vi "Read Cooler Enqueuer.vi"(11 "Cooler Controller":refnum<class "Cooler Controller.lvclass">) -> (2 "Cooler Enqueuer":refnum<class "Message Enqueuer.lvclass">)   [LabVIEW 2018, in "Cooler Controller.lvlib" / "Cooler Controller.lvclass"]
doc: "This VI reads what cooler the controller is controlling. This VI may return a Not A Refnum enqueuer because there is no guarantee that the controller is in control of any cooler."
uses:
  Cooler Controller.lvclass
  <vilib>/ActorFramework/Message Enqueuer/Message Enqueuer.lvclass
  Cooler Controller.lvclass/Cooler Controller.ctl
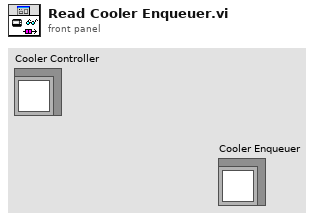
[diagram p1: front panel]
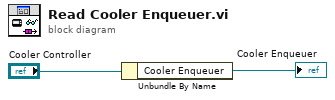
[diagram p0: block diagram]
diagram:
  n1 = Unbundle By Name("Cooler Controller") -> ("Cooler Enqueuer"=→"Cooler Enqueuer":refnum<class "Message Enqueuer.lvclass">)
